vi "Update prog list.vi"(0 "IPF files[]":T3[](array[typedef]), 1 "APG Config":T2, 2 "Inspection prog file":string, 3 "IPF cmd":T1, 4 "Programs List":i32, 5 "error in (no error)":errorcluster, 8 "data in":T4) -> (10 "data out":T4, 18 "Programs List":i32, 19 "error out":errorcluster)   [LabVIEW 2013, in "Manipulate IPF.lvlib"]
uses:
  Manipulate IPF.lvlib
  3013/code/Modules/GUI/GUI_5/subPanels/program/type_def/data.ctl
  3013/code/Modules/GUI/GUI_5/subPanels/program/type_def/Inspection program data.ctl
  3013/code/Modules/Configuration/type_def/Scan Params.ctl
  3013/code/Modules/Configuration/type_def/Profile Resolution.ctl
  3013/code/Modules/Preprocess Data/type_def/direction.ctl
  3013/code/Modules/Inspection/Data/Panel_class/type_def/Control file rel path.ctl
  3013/code/Modules/GUI/GUI_5/subPanels/edit/type_def/Description.ctl
  Pack Data/type_def/file types.ctl
  Settings/type_def/APG Config.ctl
  type_def/IPF cmd.ctl
  <vilib>/Utility/miscctls.llb/LVRowAndColumnUnsignedTypeDef.ctl
  3013/code/Modules/GUI/GUI_5/subPanels/program/program.lvlib
  Pack Data/Pack Files.lvlib
  3013/code/Modules/Configuration/Config.lvlib
  3013/code/Modules/Preprocess Data/PreProcess.lvlib
  3013/code/Modules/Inspection/Data/Panel_class/Panel.lvclass
  Settings/APG_settings.lvlib
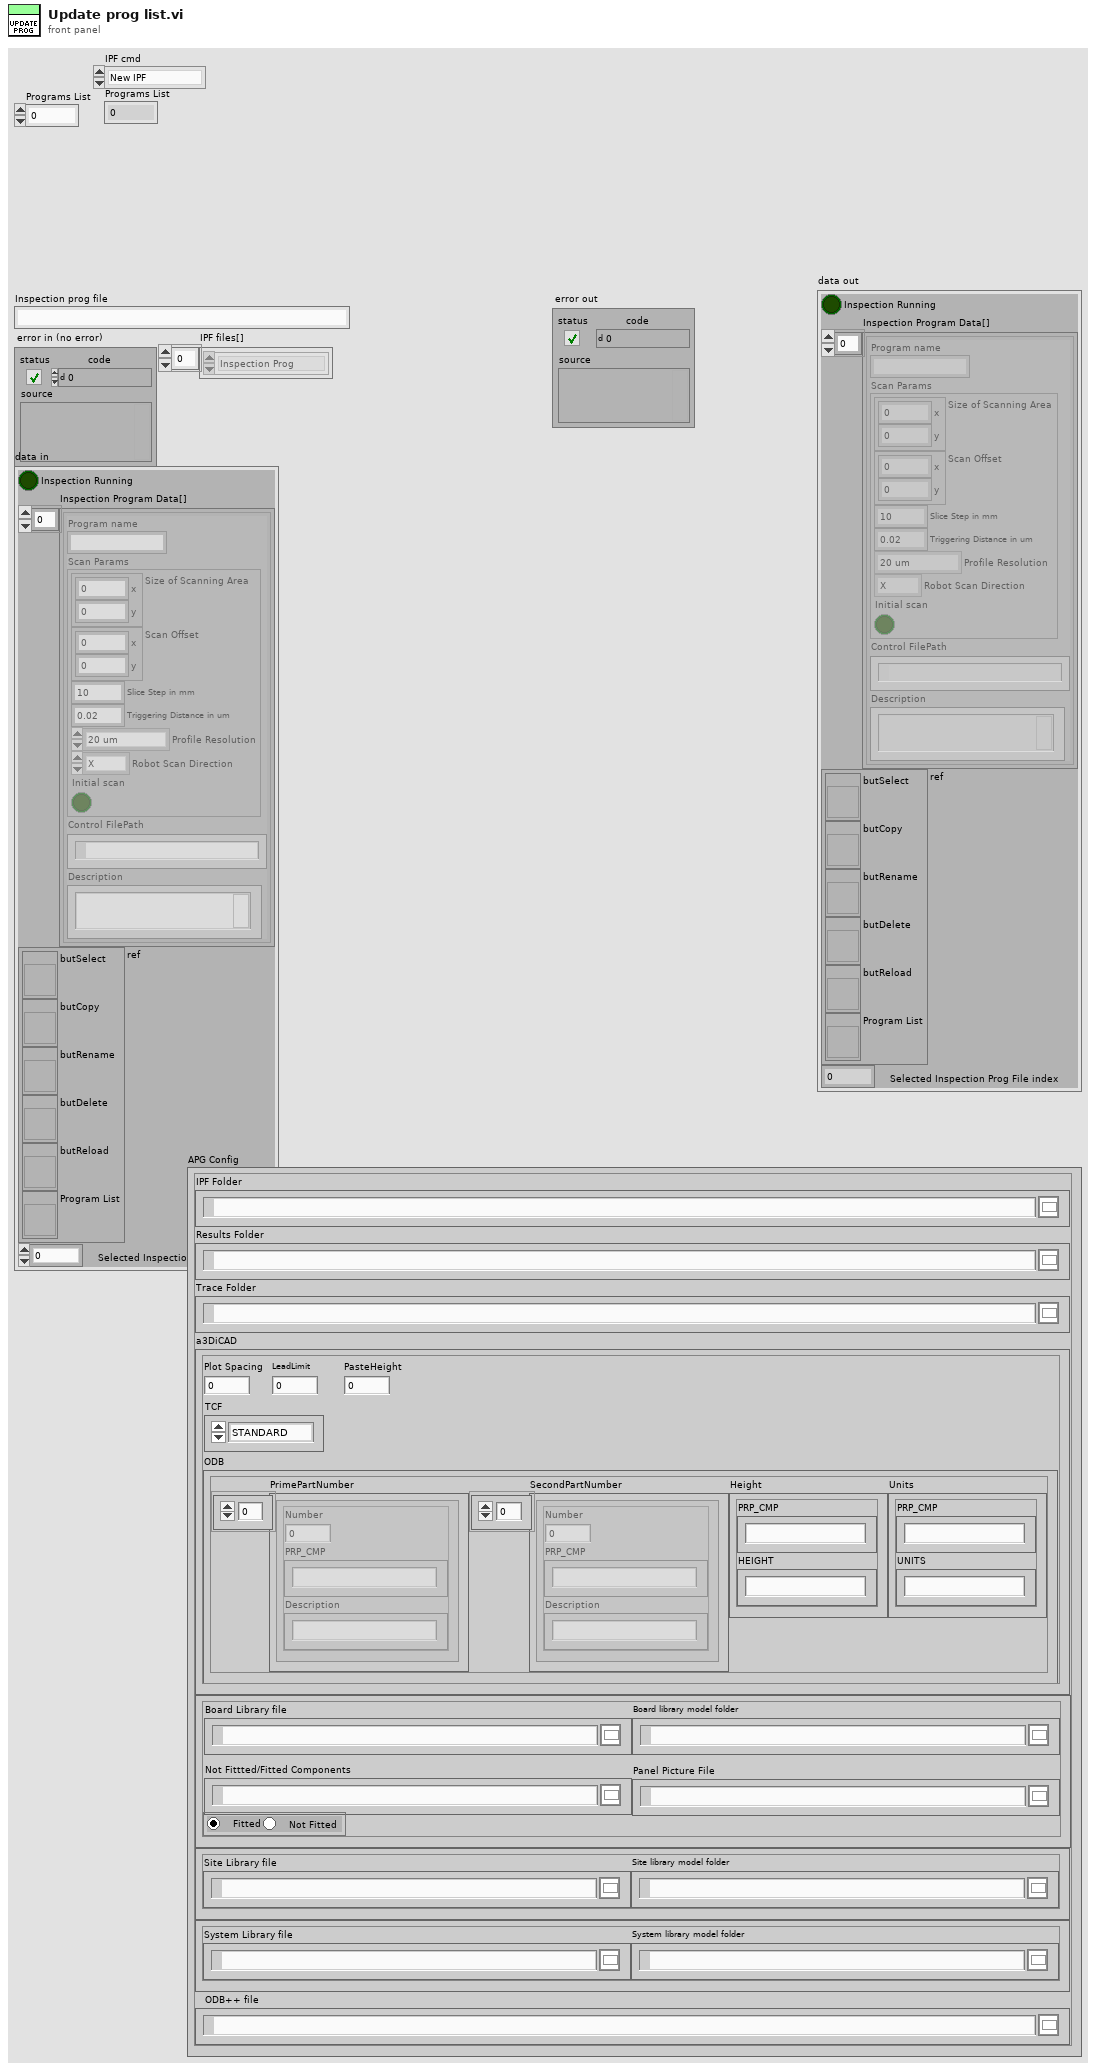
[diagram p1: front panel]
types:
  T1 = typedef "Manipulate IPF.lvlib/IPF cmd.ctl" = enum16{"New IPF", "Edit IPF", "Copy IPF", "Rename IPF", "Delete IPF", "Reload IPF", "Load all IPF"}
  T2 = typedef "APG_settings.lvlib/APG Config.ctl" = cluster{"IPF Folder":path, "Results Folder":path, "Trace Folder":path, "a3DiCAD":cluster{"Plot Spacing":dbl, "TCF":enum16{"STANDARD", "PASTE", "LEAD"}, "LeadLimit":u32, "a3DiCADDebug":bool, "ODB":cluster{"PrimePartNumber":cluster{"Number":u32, "PRP_CMP":string, "Description":string}[], "SecondPartNumber":cluster{"Number":u32, "PRP_CMP":string, "Description":string}[], "Height":cluster{"PRP_CMP":string, "HEIGHT":string}, "Units":cluster{"PRP_CMP":string, "UNITS":string}}, "PasteHeight":dbl}, "a3DiCADcfg":path, "Board Library":cluster{"Board Library file":path, "Board library model folder":path, "Not Fittted/Fitted Components":path, "Panel Picture File":path, "Components":enum32{"Fitted", "Not Fitted "}}, "Site Library":cluster{"Site Library file":path, "Site library model folder":path}, "System Library":cluster{"System Library file":path, "System library model folder":path}, "ODB++ file":path}
  T3 = typedef "Pack Files.lvlib/file types.ctl" = enum16{"ODB", "TCF", "CAD Outline", "Config", "Inspection Prog", "a3Di-bin", "Results", "CAD Labels", "CAD Pads", "calScan_fid", "calScan_cal-tab", "PCB_SerialNumber", "CAD_Assembly", "Version", "Old Results", "CAD Picture", "Old TCF"}
  T4 = typedef "GUI.lvlib/subPanel.lvlib/program.lvlib/data.ctl" = cluster{"Inspection Running":bool, "Inspection Program Data[]":T5[], "ref":cluster{"butSelect":refnum<vi>, "butCopy":refnum<vi>, "butRename":refnum<vi>, "butDelete":refnum<vi>, "butReload":refnum<vi>, "Program List":refnum<vi>}, "Selected Inspection Prog File index":i32}
  T5 = typedef "GUI.lvlib/subPanel.lvlib/program.lvlib/Inspection program data.ctl" = cluster{"Program name":string, "Scan Params":T6, "Control FilePath":T9, "Description":T10}
  T6 = typedef "Config.lvlib/Scan Params.ctl" = cluster{"Size of Scanning Area":cluster{"x":dbl, "y":dbl}, "Scan Offset":cluster{"x":dbl, "y":dbl}, "Slice Step in mm":dbl, "Triggering Distance in mm":dbl, "Triggering Distance in um":dbl, "Profile Resolution":T7, "Version":string, "Robot Scan Direction":T8, "Initial scan":bool}
  T7 = typedef "Config.lvlib/Profile Resolution.ctl" = enum8{"20 um", "40 um"}
  T8 = typedef "PreProcess.lvlib/direction.ctl" = enum8{"X", "Y"}
  T9 = typedef "Inspection.lvlib/Panel.lvclass/Control file rel path.ctl" = path
  T10 = typedef "Description.ctl" = string
  T11 = typedef "LVRowAndColumnUnsignedTypeDef.ctl" = cluster{"Row":u32, "Column":u32}
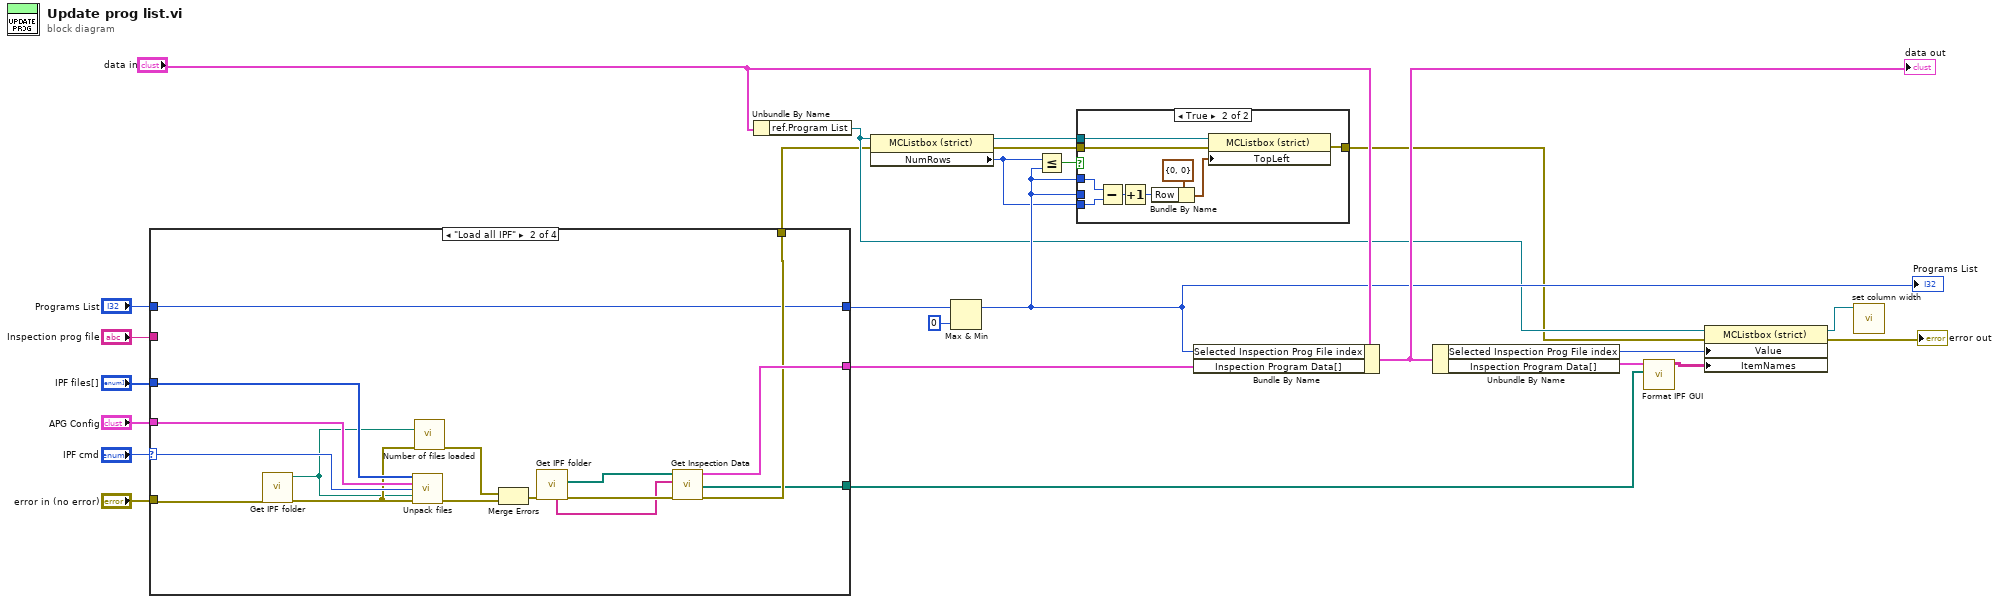
[diagram p0: block diagram]
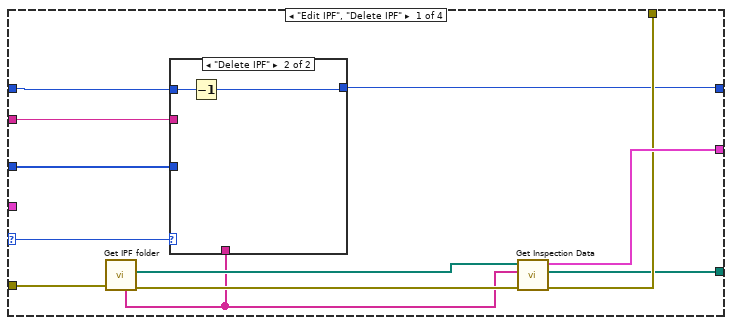
[diagram p2: hidden frame]
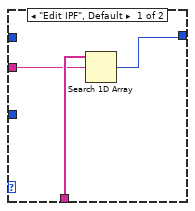
[diagram p3: hidden frame]
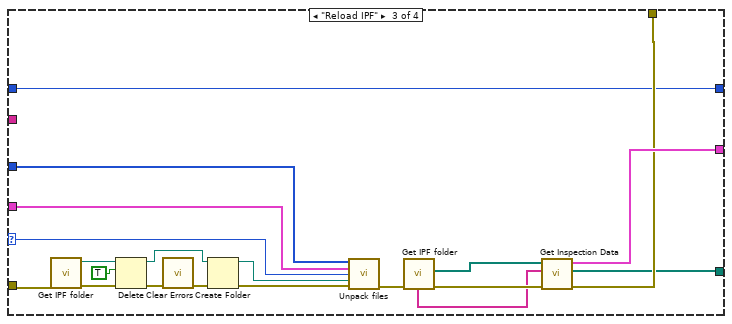
[diagram p4: hidden frame]
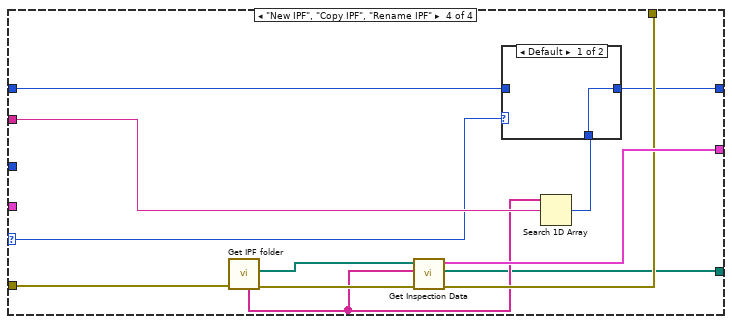
[diagram p5: hidden frame]
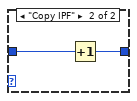
[diagram p6: hidden frame]
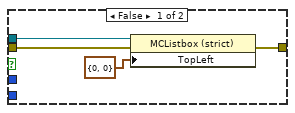
[diagram p7: hidden frame]
diagram:
  n1 = case shown="\"Load all IPF\"" "IPF cmd" {
    selector: "IPF cmd" -> [w31 w55 w75 w83]
    tunnel: [w37 w58 w78 w90] -> w15
    tunnel: "IPF files[]" -> [w30 w57 w77 _]
    tunnel: "error in (no error)" -> [w36 w54 w74 w88]
    tunnel: "Inspection prog file" -> [w29 _ _ w85]
    tunnel: [w35 w53 w73 w89] -> w3
    tunnel: "APG Config" -> [_ w51 w72 _]
    tunnel: [w32 w52 w71 w86] -> w2
    tunnel: "Programs List" -> [w33 w52 w71 w84]
    tunnel: [w26 w43 w59 w79] -> w1
    frame "Edit IPF", "Delete IPF" {
      n2 = call "Get IPF folder.vi"("error in (no error)"=w36) -> ("error out"=w28:errorcluster, "IPF sub folders"=w34:path[], "program names"=w27:string[])  [unwired: 5 in, 3 out]
      n3 = case shown="\"Delete IPF\"" w31 {
        tunnel: w33 -> [_ w42]
        tunnel: [w40 w41] -> w32
        tunnel: w30 -> [_ _]
        tunnel: w29 -> [w38 _]
        tunnel: w27 -> [w39 _]
        frame "Edit IPF", Default {
          n4 = Search 1D Array(1D array=w39, element=w38) -> (index of element=w40:i32)  [unwired: 1 in]
        }
        frame "Delete IPF" {
          n5 = Decrement(x=w42) -> (x-1=w41:i32)
        }
      }
      n6 = call "Get Inspection Data.vi"("error in (no error)"=w28, "program names"=w27, "IPF sub folders"=w34) -> ("error out"=w35:errorcluster, "IPF sub folders"=w26:path[], "Inspection Data"=w37:T5[])  [unwired: 6 in]
    }
    frame "Load all IPF" {
      n7 = call "Get IPF folder.vi"("error in (no error)"=w54) -> ("error out"=w46:errorcluster, "IPF Folder"=w45:path)  [unwired: 5 in, 4 out]
      n8 = call "Unpack files.vi"("IPF files[]"=w57, "APG Config"=w51, "IPF cmd"=w55, "Destination folder"=w45, "error in (no error)"=w46) -> ("error out"=w49:errorcluster)  [unwired: 10 in]
      n9 = call "Number of files loaded.vi"("IPF temp Folder"=w45, "error in (no error)"=w46) -> ("error out"=w47:errorcluster)  [unwired: 13 in]
      n10 = Merge Errors(w47, w49) -> (w48:errorcluster)
      n11 = call "Get IPF folder.vi"("error in (no error)"=w48) -> ("error out"=w50:errorcluster, "IPF sub folders"=w56:path[], "program names"=w44:string[])  [unwired: 5 in, 3 out]
      n12 = call "Get Inspection Data.vi"("error in (no error)"=w50, "program names"=w44, "IPF sub folders"=w56) -> ("error out"=w53:errorcluster, "IPF sub folders"=w43:path[], "Inspection Data"=w58:T5[])  [unwired: 6 in]
    }
    frame "Reload IPF" {
      n13 = call "Get IPF folder.vi"("error in (no error)"=w74) -> ("error out"=w69:errorcluster, "IPF Folder"=w68:path)  [unwired: 5 in, 4 out]
      n14 = Delete(path (use dialog)=w68, entire hierarchy (F)=TRUE, error in=w69) -> (deleted path=w63:path, error out=w66:errorcluster)  [unwired: 2 in, 1 out]
      n15 = call <vilib>:"Clear Errors.vi"("error in (no error)"=w66) -> ("error out"=w65:errorcluster)  [unwired: 6 in]
      n16 = Create Folder(path (use dialog)=w63, error in=w65) -> (created path=w62:path, error out=w64:errorcluster)  [unwired: 1 in, 1 out]
      n17 = call "Unpack files.vi"("IPF files[]"=w77, "APG Config"=w72, "IPF cmd"=w75, "Destination folder"=w62, "error in (no error)"=w64) -> ("error out"=w61:errorcluster)  [unwired: 10 in]
      n18 = call "Get IPF folder.vi"("error in (no error)"=w61) -> ("error out"=w70:errorcluster, "IPF sub folders"=w76:path[], "program names"=w60:string[])  [unwired: 5 in, 3 out]
      n19 = call "Get Inspection Data.vi"("error in (no error)"=w70, "program names"=w60, "IPF sub folders"=w76) -> ("error out"=w73:errorcluster, "IPF sub folders"=w59:path[], "Inspection Data"=w78:T5[])  [unwired: 6 in]
    }
    frame "New IPF", "Copy IPF", "Rename IPF" {
      n20 = call "Get IPF folder.vi"("error in (no error)"=w88) -> ("error out"=w82:errorcluster, "IPF sub folders"=w87:path[], "program names"=w80:string[])  [unwired: 5 in, 3 out]
      n21 = call "Get Inspection Data.vi"("error in (no error)"=w82, "program names"=w80, "IPF sub folders"=w87) -> ("error out"=w89:errorcluster, "IPF sub folders"=w79:path[], "Inspection Data"=w90:T5[])  [unwired: 6 in]
      n22 = Search 1D Array(1D array=w80, element=w85) -> (index of element=w81:i32)  [unwired: 1 in]
      n23 = case shown="Default" w83 {
        tunnel: w84 -> [_ w93]
        tunnel: [w91 w92] -> w86
        tunnel: w81 -> [w91 _]
        frame Default {
        }
        frame "Copy IPF" {
          n24 = Increment(x=w93) -> (x+1=w92:i32)
        }
      }
    }
  }
  n25 = Unbundle By Name("data in") -> ("ref.Program List"=w7:refnum<vi>)
  n26 = property class="MCListbox (strict)"(reference=w7, error in=w3) -> (reference out=w13:refnum<vi>, error out=w12:errorcluster, "NumRows"=w11:u32)
  n27 = Max & Min(x=w2, y=0) -> (max(x,y)=w20:i32)  [unwired: 1 out]
  "Programs List" <- w20
  n28 = Less Or Equal?(x=w11, y=w20) -> (x <= y?=w14:bool)
  n29 = case shown="True" w14 {
    tunnel: w13 -> [w97 w106]
    tunnel: w12 -> [w96 w105]
    tunnel: w20 -> [_ _]
    tunnel: w20 -> [_ w102]
    tunnel: w11 -> [_ w101]
    tunnel: [w94 w98] -> w4
    frame False {
      n30 = property class="MCListbox (strict)"(reference=w97, error in=w96, "TopLeft"=T11 {"Row"=0, "Column"=0} ("Top Left Visible Cell")) -> (error out=w94:errorcluster)  [unwired: 1 out]
    }
    frame True {
      n31 = Subtract(x=w102, y=w101) -> (x-y=w100:u32)
      n32 = Increment(x=w100) -> (x+1=w99:u32)
      n33 = Bundle By Name(cluster=T11 {"Row"=0, "Column"=0} ("Top Left Visible Cell"), "Row"=w99) -> (w104:T11)
      n34 = property class="MCListbox (strict)"(reference=w106, error in=w105, "TopLeft"=w104) -> (error out=w98:errorcluster)  [unwired: 1 out]
    }
  }
  n35 = Bundle By Name(cluster="data in", "Selected Inspection Prog File index"=w20, "Inspection Program Data[]"=w15) -> (w24:T4)
  "data out" <- w24
  n36 = Unbundle By Name(w24) -> ("Selected Inspection Prog File index"=w8:i32, "Inspection Program Data[]"=w5:T5[])
  n37 = call "Format IPF GUI.vi"("IPF sub folders"=w1, "Inspection Program Data[]"=w5) -> ("Item names"=w6:string[][])  [unwired: 9 in]
  n38 = property class="MCListbox (strict)"(reference=w7, error in=w4, "Value"=w8, "ItemNames"=w6) -> (reference out=w9:refnum<vi>, error out=→"error out":errorcluster)
  n39 = call "set column width.vi"("Programs List"=w9) -> ()  [unwired: 10 in]
